vi "Render.vi"(8 "error in":errorcluster, 10 "Renderer in":refnum<class "Renderer.lvclass">, 11 "Class":refnum<class "Class.lvclass">) -> (0 "error out":errorcluster, 3 "Sections out":refnum<class "Section.lvclass">[](array[class]))   [LabVIEW 2021, in "TAF Proj Document Type.lvlib" / "Class.lvclass"]
uses:
  <vilib>/Wovalab/AntiDoc/Document Type/Add-ons/LabVIEW TAF Project/Class/Class.lvclass
  C:/Program Files (x86)/National Instruments/LabVIEW 2021/vi.lib/Wovalab/AntiDoc/Bloc/Bloc.lvclass
  C:/Program Files (x86)/National Instruments/LabVIEW 2021/vi.lib/Wovalab/AntiDoc/Document Type/Add-ons/LabVIEW TAF Project/Lib/Lib.lvclass
  <vilib>/Wovalab/AntiDoc/Renderer/Renderer.lvclass
  <vilib>/Wovalab/AsciiDoc for LabVIEW/Section/Section.lvclass
  <vilib>/Wovalab/AsciiDoc for LabVIEW/Diagram/Type--enum.ctl
  <vilib>/Wovalab/AntiDoc/Bloc/Bloc.lvclass/Bloc.ctl
  <vilib>/Wovalab/AntiDoc/Document Type/Add-ons/LabVIEW TAF Project/Lib/Lib.lvclass/Lib.ctl
  <vilib>/Wovalab/AntiDoc/Document Type/Add-ons/LabVIEW TAF Project/Class/Class.lvclass/Class.ctl
  <vilib>/Wovalab/AntiDoc/Renderer/Renderer.lvclass/Renderer.ctl
  <vilib>/Wovalab/AntiDoc/Renderer/Read Image Folder Path.vi
  <vilib>/Wovalab/AntiDoc/Bloc/Read Name.vi
  <vilib>/Wovalab/AntiDoc/Document Type/Add-ons/LabVIEW TAF Project/Lib/Read Description.vi
  <vilib>/Wovalab/AntiDoc/Document Type/Add-ons/LabVIEW TAF Project/Lib/Read Version.vi
  <vilib>/Wovalab/AntiDoc/Document Type/Add-ons/LabVIEW TAF Project/Class/Read Uml.vi
  <vilib>/Wovalab/AntiDoc/Document Type/Add-ons/LabVIEW TAF Project/Lib/Read Vis.vi
  <vilib>/Wovalab/AsciiDoc for LabVIEW/Paragraph/Paragraph.lvclass
  C:/Program Files (x86)/National Instruments/LabVIEW 2021/vi.lib/Wovalab/AsciiDoc for LabVIEW/Adoc-Bloc/Bloc.lvclass
  <vilib>/Wovalab/AsciiDoc for LabVIEW/Diagram/Diagram.lvclass
  <vilib>/Wovalab/AsciiDoc for LabVIEW/Section/Add Bloc (array).vi
  <vilib>/Wovalab/AntiDoc/Document Type/Add-ons/LabVIEW TAF Project/Vi/Vi.lvclass
  <vilib>/Wovalab/AntiDoc/Utilities/Utilities.lvlib
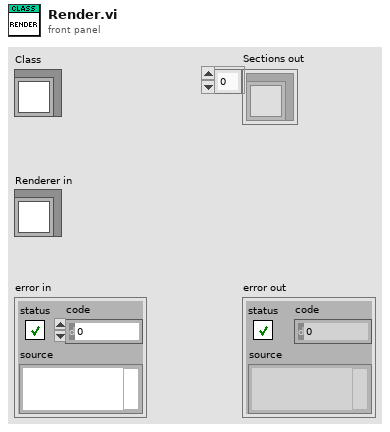
[diagram p1: front panel]
types:
  T1 = typedef "Wovalab_lib_AsciiDoctor.lvlib/Diagram.lvclass/Type--enum.ctl" = enum16{"a2s", "actdiag", "blockdiag", "ditaa", "erd", "graphviz", "meme", "mermaid", "msc", "nwdiag", "packetdiag", "plantuml", "rackdiag", "seqdiag", "shaape", "svgbob", "syntrax", "umlet", "vega", "vegalite", "wavedrom"}
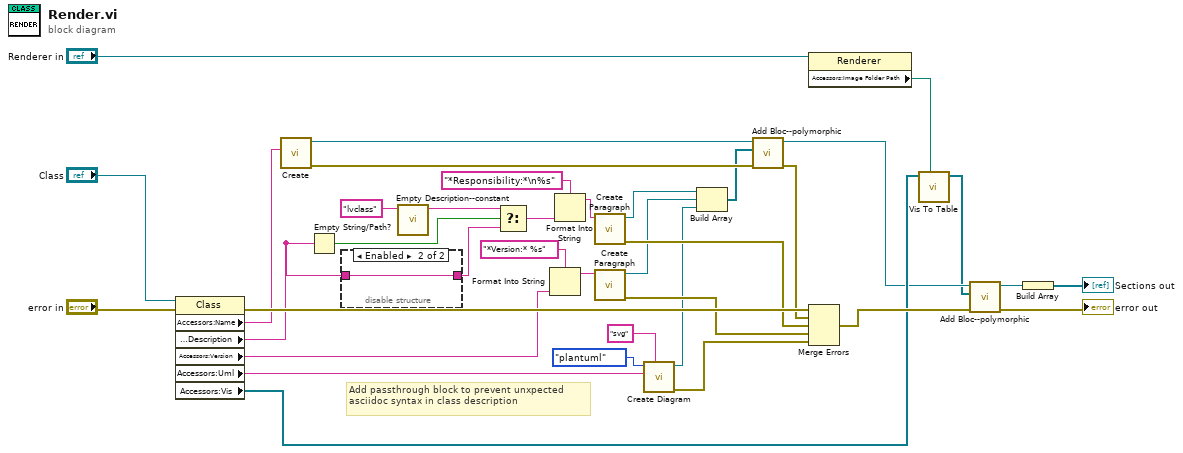
[diagram p0: block diagram]
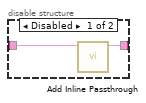
[diagram p2: hidden frame]
diagram:
  # "Add passthrough block to prevent unxpected asciidoc syntax in class description"
  n1 = property class="Class"(reference="Class", error in="error in") -> (error out=w36:errorcluster, "Accessors:Name"=w27:string, "Accessors:Description"=w1:string, "Accessors:Version"=w21:string, "Accessors:Uml"=w24:string, "Accessors:Vis"=w26:refnum<class "Vi.lvclass">[])  [unwired: 1 out]
  n2 = call <vilib>:"Create.vi"("Title"=w27) -> ("error out"=w37:errorcluster, "Section out"=w28:refnum<class "Section.lvclass">)  [unwired: 9 in]
  n3 = Empty String/Path?(string/path=w1) -> (empty?=w8:bool)
  n4 = disable-structure shown="Enabled" {
    disable-tunnel: [w39 w40] -> w2
    disable-tunnel: w1 -> [w38 w40]
    frame Disabled {
      n5 = call <vilib>:"Add Inline Passthrough.vi"("String in"=w38) -> ("String out"=w39:string)  [unwired: 10 in]
    }
    frame Enabled {
    }
  }
  n6 = call <vilib>:"Empty Description--constant.vi"("Description Source"="lvclass") -> ("Empty Description"=w3:string)  [unwired: 10 in]
  n7 = Select(t=w3, s=w8, f=w2) -> (s? t:f=w12:string)
  n8 = Format Into String(format string="*Version:* %s", w21) -> (resulting string=w15:string)  [unwired: 2 in, 1 out]
  n9 = Format Into String(format string="*Responsibility:*\n%s", w12) -> (resulting string=w13:string)  [unwired: 2 in, 1 out]
  n10 = call <vilib>:"Create Paragraph.vi"("Content"=w13) -> ("error out"=w30:errorcluster, "Paragraph out"=w10:refnum<class "Paragraph.lvclass">)  [unwired: 9 in]
  n11 = call <vilib>:"Create Paragraph.vi"("Content"=w15) -> ("error out"=w29:errorcluster, "Paragraph out"=w9:refnum<class "Paragraph.lvclass">)  [unwired: 9 in]
  n12 = call <vilib>:"Create Diagram.vi"("Format (png)"="svg", "Diagram Source Code"=w24, "Diagram Type"=Type--enum."plantuml") -> ("error out"=w32:errorcluster, "Diagram out"=w17:refnum<class "Diagram.lvclass">)  [unwired: 7 in]
  n13 = Build Array(w10, w9, w17) -> (w18:refnum<class "Bloc.lvclass">[])
  n14 = call-poly <vilib>:"Add Bloc--polymorphic.vi"("error in"=w37, "Bloc"=w18, "Section in"=w28) -> ("error out"=w31:errorcluster, "Section out"=w23:refnum<class "Section.lvclass">)  [unwired: 7 in]
  n15 = property class="Renderer"(reference="Renderer in") -> ("Accessors:Image Folder Path"=w6:path)  [unwired: 1 in, 2 out]
  n16 = Merge Errors(w36, w31, w30, w29, w32) -> (w35:errorcluster)
  n17 = call <vilib>:"Vis To Table.vi"("Image Folder Path"=w6, "Vis"=w26) -> ("Table"=w7:refnum<class "Bloc.lvclass">[])  [unwired: 9 in]
  n18 = call-poly <vilib>:"Add Bloc--polymorphic.vi"("error in"=w35, "Bloc"=w7, "Section in"=w23) -> ("error out"=→"error out":errorcluster, "Section out"=w20:refnum<class "Section.lvclass">)  [unwired: 7 in]
  n19 = Build Array(w20) -> (→"Sections out":refnum<class "Section.lvclass">[])
